vi "脉冲脚本.vi"(1 "4-wire":bool, 2 "脉冲":T1 {"测试参数"."反向极限电流(mA)" min=0.0 max=3000.0; "测试参数"."反向电压(V)" min=0.0 max=40.0; "测试参数"."读取电压(V)" min=0.0 max=40.0; "测试参数"."正向极限电流(mA)" min=0.0 max=3000.0; "测试参数"."正向电压(V)" min=0.0 max=40.0}, 3 "方向(T:正向)":bool=TRUE) -> (0 "Script":string)   [LabVIEW 2021]
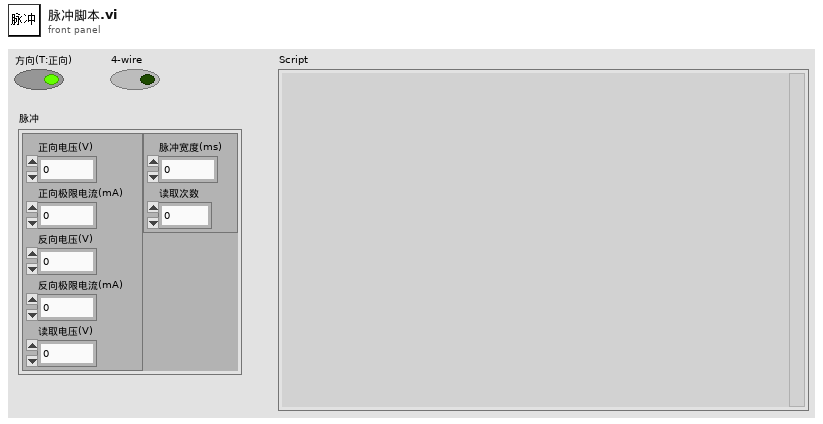
[diagram p1: front panel]
types:
  T1 = typedef "脉冲参数.ctl" = cluster{"测试参数":cluster{"正向电压(V)":dbl, "正向极限电流(mA)":dbl, "反向电压(V)":dbl, "反向极限电流(mA)":dbl, "读取电压(V)":dbl}, "时序参数":cluster{"脉冲宽度(ms)":dbl, "读取次数":u32}}
  T2 = cluster{"正向电压(V)":dbl, "正向极限电流(mA)":dbl, "反向电压(V)":dbl, "反向极限电流(mA)":dbl, "读取电压(V)":dbl}
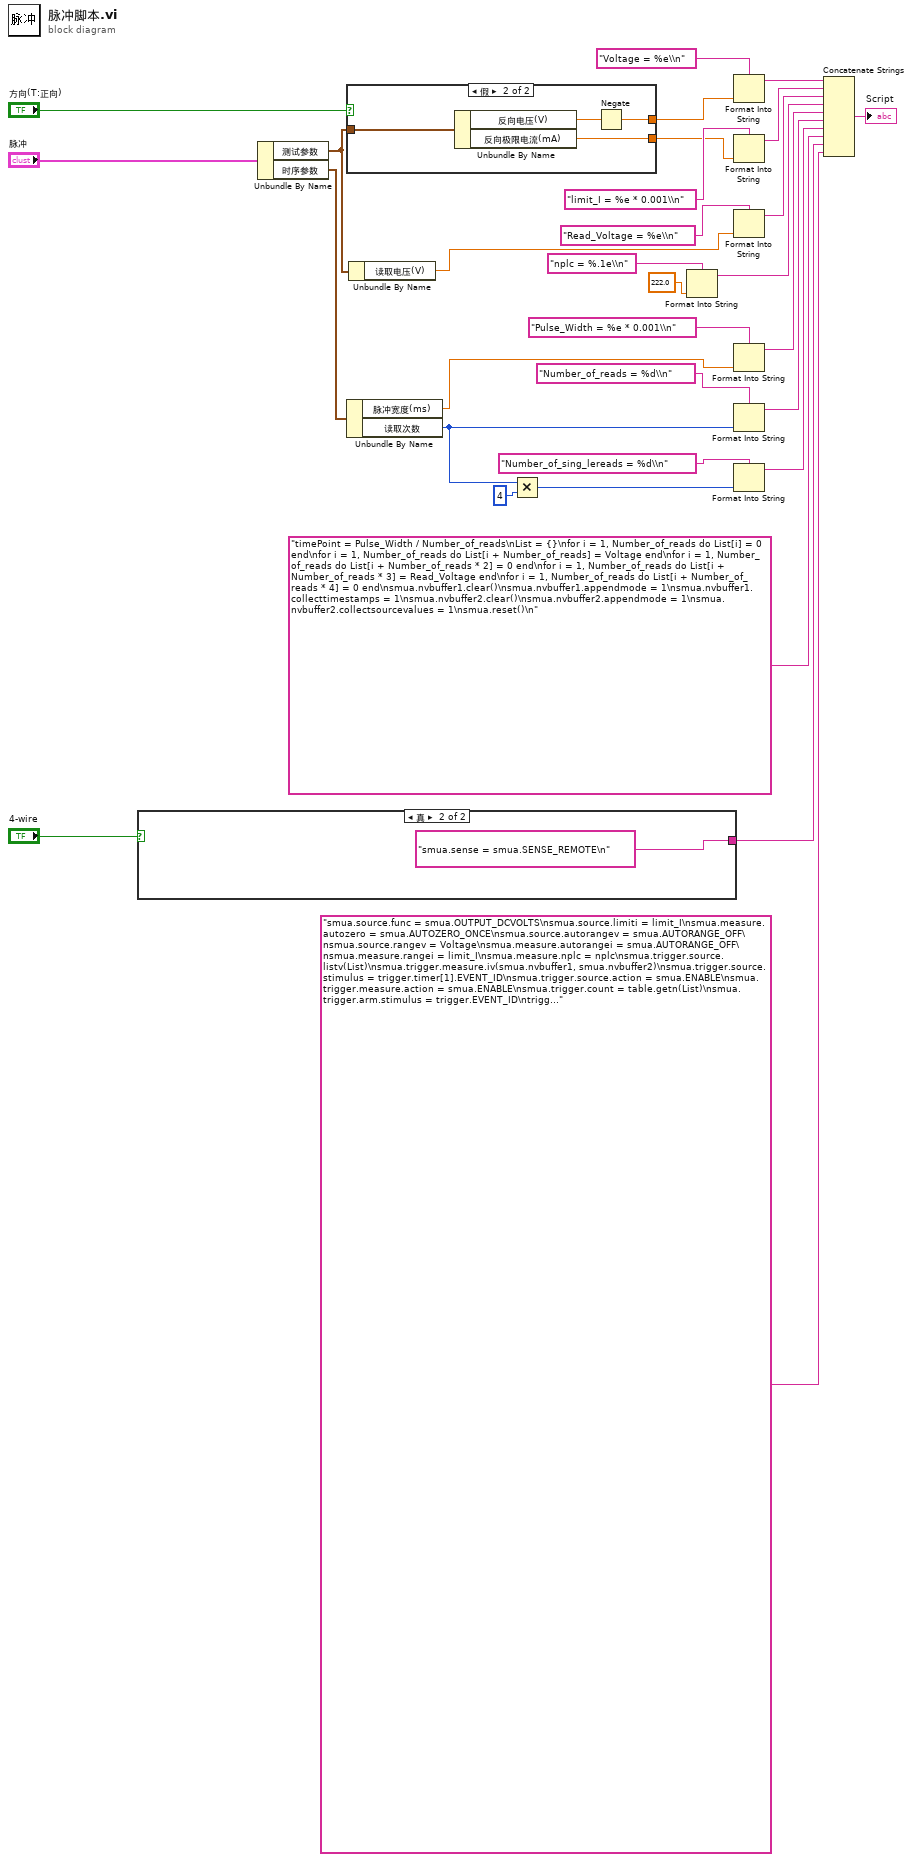
[diagram p0: block diagram]
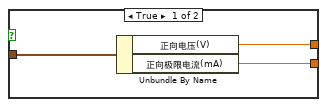
[diagram p2: hidden frame]
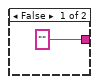
[diagram p3: hidden frame]
diagram:
  n1 = case shown="真" "4-wire" {
    tunnel: ["" "smua.sense = smua.SENSE_REMOTE\n"] -> w23
    frame False {
    }
    frame True {
    }
  }
  n2 = Unbundle By Name("脉冲") -> ("测试参数"=w10:T2, "时序参数"=w8:cluster{"脉冲宽度(ms)":dbl, "读取次数":u32})
  n3 = case shown="假" "方向(T:正向)" {
    tunnel: w10 -> [w36 w40]
    tunnel: [w35 w37] -> w12
    tunnel: [w34 w39] -> w11
    frame True {
      n4 = Unbundle By Name(w36) -> ("正向电压(V)"=w35:dbl, "正向极限电流(mA)"=w34:dbl)
    }
    frame False {
      n5 = Unbundle By Name(w40) -> ("反向电压(V)"=w38:dbl, "反向极限电流(mA)"=w39:dbl)
      n6 = Negate(x=w38) -> (-x=w37:dbl)
    }
  }
  n7 = Unbundle By Name(w8) -> ("脉冲宽度(ms)"=w7:dbl, "读取次数"=w4:u32)
  n8 = Unbundle By Name(w10) -> ("读取电压(V)"=w9:dbl)
  n9 = Multiply(x=w4, y=u32 4) -> (x*y=w17:u32)
  n10 = Format Into String(format string="nplc = %.1e\\n", 222.0 ("输入 1")) -> (resulting string=w1:string)  [unwired: 2 in, 1 out]
  n11 = Format Into String(format string="Voltage = %e\\n" ("格式字符串"), w12) -> (resulting string=w28:string)  [unwired: 2 in, 1 out]
  n12 = Format Into String(format string="limit_I = %e * 0.001\\n" ("格式字符串"), w11) -> (resulting string=w14:string)  [unwired: 2 in, 1 out]
  n13 = Format Into String(format string="Read_Voltage = %e\\n" ("格式字符串"), w9) -> (resulting string=w13:string)  [unwired: 2 in, 1 out]
  n14 = Format Into String(format string="Pulse_Width = %e * 0.001\\n", w7) -> (resulting string=w2:string)  [unwired: 2 in, 1 out]
  n15 = Format Into String(format string="Number_of_reads = %d\\n" ("格式字符串"), w4) -> (resulting string=w19:string)  [unwired: 2 in, 1 out]
  n16 = Format Into String(format string="Number_of_sing_lereads = %d\\n" ("格式字符串"), w17) -> (resulting string=w18:string)  [unwired: 2 in, 1 out]
  n17 = Concatenate Strings(w28, w14, w13, w1, w2, w19, w18, "timePoint = Pulse_Width / Number_of_reads\nList = {}\nfor i = 1, Number_of_reads do List[i] = 0 end\nfor i = 1, Number_of_reads do List[i + Number_of_reads] = Voltage end\nfor i = 1, Number_of_reads do List[i + Number_of_reads * 2] = 0 end\nfor i = 1, Number_of_reads do List[i + Number_of_reads * 3] = Read_Voltage end\nfor i = 1, Number_of_reads do List[i + Number_of_reads * 4] = 0 end\nsmua.nvbuffer1.clear()\nsmua.nvbuffer1.appendmode = 1\nsmua.nvbuffer1.collecttimestamps = 1\nsmua.nvbuffer2.clear()\nsmua.nvbuffer2.appendmode = 1\nsmua.nvbuffer2.collectsourcevalues = 1\nsmua.reset()\n", w23, "smua.source.func = smua.OUTPUT_DCVOLTS\nsmua.source.limiti = limit_I\nsmua.measure.autozero = smua.AUTOZERO_ONCE\nsmua.source.autorangev = smua.AUTORANGE_OFF\nsmua.source.rangev = Voltage\nsmua.measure.autorangei = smua.AUTORANGE_OFF\nsmua.measure.rangei = limit_I\nsmua.measure.nplc = nplc\nsmua.trigger.source.listv(List)\nsmua.trigger.measure.iv(smua.nvbuffer1, smua.nvbuffer2)\nsmua.trigger.source.stimulus = trigger.timer[1].EVENT_ID\nsmua.trigger.source.action = smua.ENABLE\nsmua.trigger.measure.action = smua.ENABLE\nsmua.trigger.count = table.getn(List)\nsmua.trigger.arm.stimulus = trigger.EVENT_ID\ntrigger.timer[1].reset()\ntrigger.timer[1].stimulus = smua.trigger.ARMED_EVENT_ID\ntrigger.timer[1].passthrough = false\ntrigger.timer[1].delay = timePoint\ntrigger.timer[1].count = table.getn(List)\nsmua.source.output = smua.OUTPUT_ON\nsmua.trigger.initiate()\ndelay(1e-3)\nsmua.trigger.arm.set()\nfunction _done()\n    Start = 1\n    Stop = Number_of_sing_lereads\n    repeat\n        if (bit.test(status.operation.instrument.smua.condition, 4) == false) then\n            smua.source.leveli = 0\n            smua.source.levelv = 0\n            smua.source.output = smua.OUTPUT_OFF\n            Stop = table.getn(List)\n            print(\"{\" .. Stop - Start + 1 .. \"}\")\n            printbuffer(Start, Stop, smua.nvbuffer1.timestamps)\n            printbuffer(Start, Stop, smua.nvbuffer2.sourcevalues)\n            printbuffer(Start, Stop, smua.nvbuffer1)\n            printbuffer(Start, Stop, smua.nvbuffer2)\n            print(\"{done}\")\n            return\n        elseif (smua.nvbuffer1.n > Stop) then\n            print(\"{\" .. Number_of_sing_lereads .. \"}\")\n            printbuffer(Start, Stop, smua.nvbuffer1.timestamps)\n            printbuffer(Start, Stop, smua.nvbuffer2.sourcevalues)\n            printbuffer(Start, Stop, smua.nvbuffer1)\n            printbuffer(Start, Stop, smua.nvbuffer2)\n            Start = Start + Number_of_sing_lereads\n            Stop = Stop + Number_of_sing_lereads\n        end\n        delay(timePoint)\n    until (false)\nend\n_done()\nreset()\n") -> (→"Script":string)
